vi "FRIC_navX_Get_YPRHfH.vi"(5 "Device Number":T1, 6 "Zero":bool, 7 "Update":bool) -> (2 "YRPHfH":T2)   [LabVIEW 2015]
doc: "This navX VI returns the Yaw, Roll, Pitch, Heading, Fused Heading of the navX."
uses:
  _TypeDefs/FRIC_navX_DeviceNumbersTypeDef.ctl
  _TypeDefs/Z900_navX_DeviceRegisters.ctl
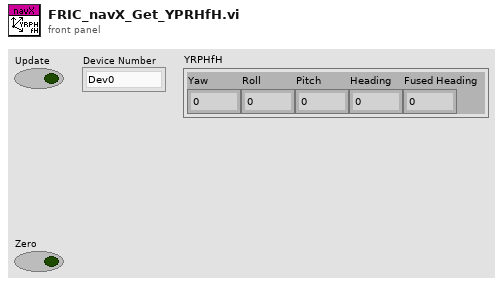
[diagram p1: front panel]
types:
  T1 = typedef "FRIC_navX_DeviceNumbersTypeDef.ctl" = enum16{"Dev0", "Dev1", "Dev2", "Dev3", "Dev4", "Dev5", "Dev6", "Dev7", "Dev8", "Dev9", "Dev10"}
  T2 = cluster{"Yaw":dbl, "Roll":dbl, "Pitch":dbl, "Heading":dbl, "Fused Heading":dbl}
  T3 = typedef "Z900_navX_DeviceRegisters.ctl" = u8
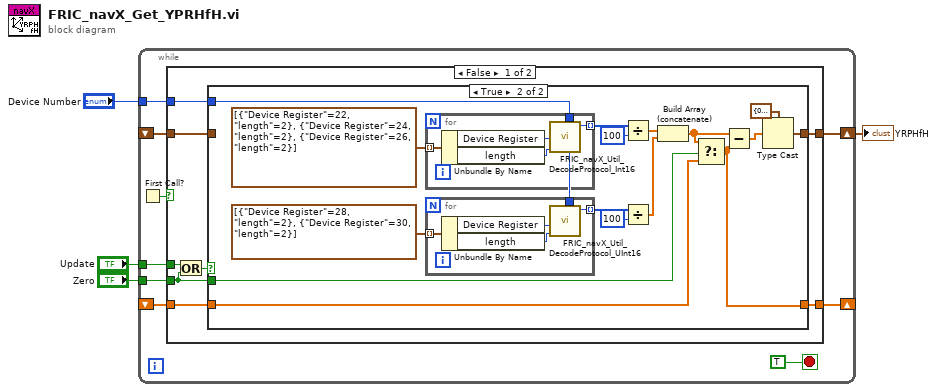
[diagram p0: block diagram]
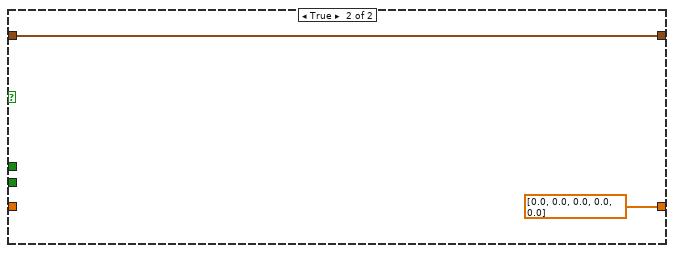
[diagram p3: hidden frame]
diagram:
  n1 = while {
    shift-right: [w11] -> w4
    shift-left: _ -> [w12]
    tunnel: "Update" -> [w10]
    shift-right: [w8] -> _
    shift-left: _ -> [w9]
    tunnel: "Zero" -> [w7]
    tunnel: "Device Number" -> [w5]
    stop <- TRUE stop-if-true
    n2 = First Call?() -> (First Call?: T/F=w6:bool)
    n3 = case shown="False" w6 {
      tunnel: w12 -> [w21 w51]
      tunnel: [w20 w51] -> w11
      tunnel: w10 -> [w17 _]
      tunnel: w9 -> [w19 _]
      tunnel: [w18 dbl[] [0.0, 0.0, 0.0, 0.0, 0.0] ("f")] -> w8
      tunnel: w7 -> [w16 _]
      tunnel: w5 -> [w14 _]
      frame False {
        n4 = Or(x=w17, y=w16) -> (x .or. y?=w15:bool)
        n5 = case shown="True" w15 {
          tunnel: [w23 w38] -> w20
          tunnel: w21 -> [w23 _]
          tunnel: w19 -> [w22 w27]
          tunnel: [w22 w26] -> w18
          tunnel: w16 -> [_ w25]
          tunnel: w14 -> [_ w24]
          frame False {
          }
          frame True {
            n6 = for {
              tunnel: cluster{"Device Register":T3, "length":i32}[] [{"Device Register"=22, "length"=2}, {"Device Register"=24, "length"=2}, {"Device Register"=26, "length"=2}] ("Array") -> [w47] mode=indexing
              tunnel: [w46] -> w33 mode=indexing
              tunnel: w24 -> [w45]
              n7 = Unbundle By Name(w47) -> ("Device Register"=w49:T3, "length"=w48:i32)
              n8 = call "FRIC_navX_Util_DecodeProtocol_Int16.vi"("Device Number"=w45, "length"=w48, "Device Register"=w49) -> ("Value"=w46:i16)  [unwired: 8 in]
            }
            n9 = for {
              tunnel: cluster{"Device Register":T3, "length":i32}[] [{"Device Register"=28, "length"=2}, {"Device Register"=30, "length"=2}] ("Array") -> [w44] mode=indexing
              tunnel: [w41] -> w31 mode=indexing
              tunnel: w24 -> [w40]
              n10 = Unbundle By Name(w44) -> ("Device Register"=w43:T3, "length"=w42:i32)
              n11 = call "FRIC_navX_Util_DecodeProtocol_UInt16.vi"("Device Number"=w40, "length"=w42, "Device Register"=w43) -> ("Value"=w41:u16)  [unwired: 8 in]
            }
            n12 = Divide(x=w33, y=100) -> (x/y=w30:dbl[])
            n13 = Divide(x=w31, y=100) -> (x/y=w35:dbl[])
            n14 = Build Array (concatenate)(w30, w35) -> (w28:dbl[])
            n15 = Select(t=w28, s=w25, f=w27) -> (s? t:f=w26:dbl[])
            n16 = Subtract(x=w28, y=w26) -> (x-y=w29:dbl[])
            n17 = Type Cast(type=T2 {"Yaw"=0.0, "Roll"=0.0, "Pitch"=0.0, "Heading"=0.0, "Fused Heading"=0.0}, x=w29) -> (*(type *) &x=w38:T2)
          }
        }
      }
      frame True {
      }
    }
  }
  "YRPHfH" <- w4
